vi "add_num_float_to_send_frame_7.vi"(10 "num_float":sgl, 11 "id (2 characters)":string) -> (3 "String":string)   [LabVIEW 2020]
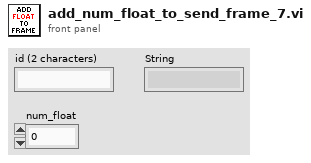
[diagram p1: front panel]
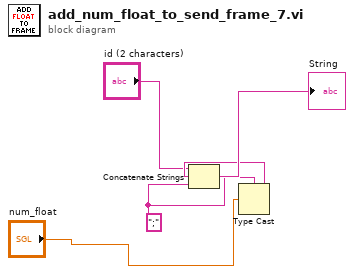
[diagram p0: block diagram]
diagram:
  w3 = ";" ("string")
  n1 = Type Cast(type=w3, x="num_float") -> (*(type *) &x=w2:string)
  n2 = Concatenate Strings("id (2 characters)", w2, w3) -> (→"String":string)
